vi "combo_box_string_write.vi"() -> ()   [LabVIEW 2010]
panel:
  in  "Cluster":cluster{"Combo Box":string}
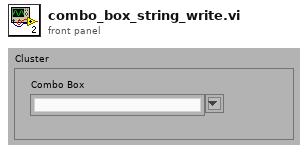
[diagram p1: front panel]
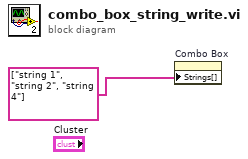
[diagram p0: block diagram]
diagram:
  n1 = property on="Combo Box" class="CmbBox"("Strings[]"=string[] ["string 1", "string 2", "string 4"]) -> ()  [unwired: 2 in, 2 out]
